vi "NMRfast.vi"() -> ()   [LabVIEW 2013]
uses:
  <vilib>/Utility/file.llb/Read From Spreadsheet File (DBL).vi
  <vilib>/Analysis/NI_AALBase.lvlib
panel:
  out "Diff Sigma":dbl format="%#_13g"
  out "Peak center (MHz)":sgl=213.01303 format="%.3f"
  out "Peak width (MHz)":sgl=0.03243152 format="%.5f"
  in  "Max":bool
  in  "Logoffset (V)":dbl=-5.996000000000003 min=-9.0 max=0.0 step=0.0005 format="%_5g"
  in  "Phase (V)":dbl=6.500000000000002 min=0.0 max=9.0 step=0.0005 format="%_5g"
  out "Telnet error out":errorcluster
  in  "Real/Quad Q curve":bool=TRUE
  out "Temperature (C)":dbl(graph)=26.25
  out "+3V supply":dbl=3.245 format="%_4g"
  out "Temp (C)":dbl=26.25 format="%_4g"
  in  "RemovePed":bool=TRUE
  in  "IF / LOG Det":bool
  in  "Q curve file":string="realback212a.txt"
  out "File name 2":string="C:\\users\\plm\\Desktop\\rssmt\\realback212a.txt"
  in  "AutoTune":bool
  out "RF OK":bool=TRUE
  out "Peak area (V-MHz)":sgl=0.0029111227 format="%.5f"
  in  "Gauss Fit":bool
  out "NMR Graph + Fit":cluster{cluster{dbl, "Numeric":dbl}[]}[](graph)=[{[{212.6, "Numeric"=-0.0034599166666668653}, {212.60999999999999, "Numeric"=-0.0019199166666681458}, {212.62, "Numeric"=-0.0024159166666654327}, {212.63, "Numeric"=-0.0024479166666666894}, {212.64, "Numeric"=-0.002915916666667886}, {212.65, "Numeric"=-0.003319916666665379}, {212.66, "Numeric"=-0.0013599166666665415}, {212.67, "Numeric"=-0.0008359166666676411}, {212.68, "Numeric"=-0.000347916666665349}, {212.69, "Numeric"=-0.00019591666666641475}, {212.7, "Numeric"=-0.0012799166666674225}, {212.71, "Numeric"=-0.001799916666665344}, {212.72, "Numeric"=-0.00205591666666632}, {212.73, "Numeric"=-0.0023479166666672295}, {212.74, "Numeric"=-0.0016759166666680753}, {212.75, "Numeric"=-0.0010399166666662475}, {212.76, "Numeric"=-0.0017399166666670638}, {212.77, "Numeric"=-0.0017759166666678145}, {212.78, "Numeric"=-4.7916666666199086e-05}, {212.79, "Numeric"=-0.000755916666666921}, {212.8, "Numeric"=-0.0004999166666675783}, {212.81, "Numeric"=-0.000479916666666174}, {212.82, "Numeric"=0.00010408333333319572}, {212.82999999999998, "Numeric"=5.208333333263284e-05}, {212.84, "Numeric"=0.0012640833333338224}, {212.85, "Numeric"=0.001440083333333288}, {212.85999999999999, "Numeric"=0.00018008333333281723}, {212.87, "Numeric"=-0.0004159166666662063}, {212.88, "Numeric"=0.00015208333333335388}, {212.89, "Numeric"=-0.0004159166666670216}, {212.9, "Numeric"=8.008333333374331e-05}, {212.91, "Numeric"=0.0012400833333333942}, {212.92, "Numeric"=0.001664083333333114}, {212.93, "Numeric"=0.0014520833333336643}, {212.94, "Numeric"=0.003104083333333411}, {212.95, "Numeric"=0.005720083333333222}, {212.96, "Numeric"=0.01040008333333356}, {212.97, "Numeric"=0.019844083333333404}, {212.98, "Numeric"=0.030252083333333308}, {212.99, "Numeric"=0.03002408333333328}, {213.0, "Numeric"=0.02346008333333337}, {213.01, "Numeric"=0.01956008333333337}, {213.02, "Numeric"=0.017724083333333435}, {213.03, "Numeric"=0.014152083333333312}, {213.04, "Numeric"=0.014044083333333405}, {213.05, "Numeric"=0.015100083333333562}, {213.06, "Numeric"=0.015320083333333224}, {213.07, "Numeric"=0.01620408333333341}, {213.08, "Numeric"=0.013052083333333665}, {213.09, "Numeric"=0.009264083333333114}, {213.1, "Numeric"=0.006440083333333396}, {213.11, "Numeric"=0.005480083333333742}, {213.12, "Numeric"=0.005284083333332979}, {213.13, "Numeric"=0.004852083333333353}, {213.14000000000001, "Numeric"=0.0034840833333337944}, {213.15, "Numeric"=0.002580083333332819}, {213.16, "Numeric"=0.0032400833333332884}, {213.17000000000002, "Numeric"=0.004064083333333823}, {213.18, "Numeric"=0.003452083333332633}, {213.19, "Numeric"=0.003604083333333198}, {213.2, "Numeric"=0.003520083333333825}, {213.21, "Numeric"=0.003500083333332421}, {213.22, "Numeric"=0.0018440833333330771}, {213.23, "Numeric"=0.0016520833333337993}, {213.24, "Numeric"=0.0013240833333345902}, {213.25, "Numeric"=0.00026008333333293627}, {213.26, "Numeric"=0.000760083333333752}, {213.27, "Numeric"=0.0010240833333346388}, {213.28, "Numeric"=0.0006520833333327732}, {213.29, "Numeric"=0.0013440833333336804}, {213.3, "Numeric"=0.0012000833333346552}, {213.31, "Numeric"=0.001420083333332575}, {213.32, "Numeric"=0.0020040833333335823}, {213.33, "Numeric"=0.0020520833333346504}, {213.34, "Numeric"=-0.00013591666666763844}, {213.35, "Numeric"=-0.0009599166666665439}, {213.36, "Numeric"=-0.0002199166666653771}, {213.37, "Numeric"=-0.0004159166666678838}, {213.38, "Numeric"=0.00045208333333330696}, {213.39000000000001, "Numeric"=0.0012840833333345658}, {213.4, "Numeric"=0.0008800833333318511}]}]
  in  "Amp of Q curve":dbl=1.8000000000000034 min=0.0 max=29.0 step=0.01 format="%_3f"
  in  "Subtract Q curve":bool=TRUE
  out "Pedestal Offset":dbl(graph)=0.006135416666666641
  out "Pedestal Difference":dbl(graph)=0.002880166666666909
  out "# Good Spectra":i32=988
  in  "Quality cuts":bool=TRUE
  out "Pedestal OK":bool=TRUE
  out "Sweep #":i32=10
  out "1st Sweep":bool
  out "ADC volts OK":bool=TRUE
  out "Peak Height Distribution":cluster{"Y":dbl[], "Y":dbl[]}[](graph)=[{"Y"=[0.02747215624999998, 0.027537302083333312, 0.027602447916666644, 0.02766759374999998, 0.02773273958333331, 0.027797885416666647, 0.02786303124999998, 0.02792817708333331, 0.027993322916666646, 0.02805846874999998, 0.028123614583333314, 0.028188760416666646, 0.028253906249999978, 0.028319052083333313, 0.028384197916666645, 0.02844934374999998, 0.028514489583333313, 0.028579635416666645, 0.02864478124999998, 0.028709927083333312, 0.028775072916666644, 0.02884021874999998, 0.02890536458333331, 0.028970510416666647, 0.02903565624999998, 0.02910080208333331, 0.029165947916666646, 0.02923109374999998, 0.029296239583333314, 0.029361385416666646, 0.029426531249999978, 0.029491677083333313, 0.029556822916666645, 0.02962196874999998, 0.029687114583333313, 0.029752260416666645, 0.02981740624999998, 0.029882552083333312, 0.029947697916666648, 0.03001284374999998, 0.03007798958333331, 0.030143135416666647, 0.03020828124999998, 0.03027342708333331, 0.030338572916666647, 0.03040371874999998, 0.030468864583333314, 0.030534010416666646, 0.030599156249999978, 0.030664302083333313, 0.030729447916666645, 0.03079459374999998, 0.030859739583333313, 0.030924885416666645, 0.03099003124999998, 0.031055177083333312, 0.031120322916666648, 0.03118546874999998, 0.031250614583333315, 0.031315760416666644, 0.03138090624999998, 0.031446052083333315, 0.03151119791666664, 0.03157634374999998, 0.031641489583333314, 0.03170663541666665, 0.03177178124999998, 0.03183692708333331, 0.03190207291666665, 0.03196721874999998, 0.03203236458333331, 0.03209751041666665, 0.03216265624999998, 0.03222780208333331, 0.03229294791666665, 0.032358093749999976, 0.03242323958333331, 0.03248838541666665, 0.03255353124999998, 0.03261867708333331, 0.03268382291666665, 0.03274896874999998, 0.03281411458333331, 0.032879260416666646, 0.03294440624999998, 0.03300955208333331, 0.033074697916666645, 0.03313984374999998, 0.033204989583333316, 0.033270135416666645, 0.03333528124999998, 0.033400427083333316, 0.033465572916666644, 0.03353071874999998, 0.033595864583333315, 0.033661010416666644, 0.03372615624999998, 0.033791302083333315, 0.03385644791666664, 0.03392159374999998], "Y"=[4.0, 0.0, 0.0, 0.0, 2.0, 1.0, 4.0, 2.0, 4.0, 1.0, 2.0, 3.0, 2.0, 6.0, 3.0, 2.0, 4.0, 7.0, 5.0, 5.0, 11.0, 4.0, 7.0, 6.0, 10.0, 7.0, 10.0, 6.0, 14.0, 16.0, 11.0, 9.0, 13.0, 10.0, 12.0, 17.0, 20.0, 12.0, 18.0, 10.0, 15.0, 13.0, 11.0, 19.0, 21.0, 12.0, 18.0, 21.0, 23.0, 16.0, 24.0, 15.0, 12.0, 17.0, 18.0, 26.0, 22.0, 26.0, 29.0, 17.0, 29.0, 20.0, 16.0, 14.0, 13.0, 13.0, 16.0, 19.0, 12.0, 13.0, 16.0, 6.0, 9.0, 9.0, 11.0, 9.0, 5.0, 9.0, 9.0, 2.0, 10.0, 4.0, 11.0, 10.0, 3.0, 5.0, 3.0, 4.0, 3.0, 6.0, 2.0, 2.0, 3.0, 1.0, 1.0, 4.0, 4.0, 3.0, 1.0, 3.0]}]
  in  "# of Sweeps":i32=1000
  out "S/N":dbl=24.050317766918518 format="%_3g"
  out "Peak mean (V)":dbl=0.030799925016869054 format="%_4g"
  out "Peak Height":dbl(graph)=0.030252083333333308
  in  "Raw Data":bool=TRUE
  in  "Tank RF":bool=TRUE
  in  "IF Atten (dB)":i8=3 min=0 max=31 step=1
  in  "IFoffset (V)":dbl=5.2303410000000135 min=-0.0 max=9.0 step=0.001 format="%.4f"
  in  "Tune  (V)":dbl=0.3670000000000009 min=-0.5 max=8.0 step=0.001 format="%.4f"
  in  "Hi / Lo Gain":bool
  out "Voltage Array":sgl[](array[numeric])=[0.0322, 0.0323, 0.0304, 0.029, 0.0272, 0.0255, 0.0262, 0.0255, 0.0248, 0.0238, 0.0216, 0.02, 0.0187, 0.0174, 0.0171, 0.0168, 0.0152, 0.0143, 0.0152, 0.0137, 0.0132, 0.0125, 0.0124, 0.0117, 0.0123, 0.0119, 0.0101, 0.009, 0.0091, 0.0081, 0.0082, 0.009, 0.0091, 0.0086, 0.01, 0.0124, 0.0169, 0.0262, 0.0365, 0.0362, 0.0296, 0.0257, 0.0239, 0.0204, 0.0204, 0.0216, 0.022, 0.0231, 0.0202, 0.0167, 0.0142, 0.0136, 0.0138, 0.0138, 0.0129, 0.0125, 0.0137, 0.0151, 0.0151, 0.0159, 0.0165, 0.0172, 0.0163, 0.0169, 0.0174, 0.0172, 0.0186, 0.0198, 0.0204, 0.0221, 0.023, 0.0243, 0.026, 0.0272, 0.0262, 0.0266, 0.0286, 0.0297, 0.0319, 0.0341, 0.0351] format="%.4f"
  in  "Invert Polarity":bool=TRUE
  out "Pedestal Diff (V)":sgl=0.0028801668 format="%.3f"
  out "Peak amp (V)":sgl=0.030252084 format="%.3f"
  in  "Save Data to File":bool
  in  "RF Level (dBm)":dbl min=-10.0 max=10.0 step=0.1 format="%.2f"
  out "SMT error out":errorcluster
  out "Sample RMS (V)":dbl=0.0009296296296296295 format="%.4f"
  in  "# Sample/step":i32=80 min=1 max=5000 step=100
  in  "Step Width (MHz)":dbl=0.01 min=0.0 max=1000.0 step=0.0001 format="%.4f"
  in  "Freq Span (MHz)":dbl=0.8 min=0.0 max=3000.0 step=0.1 format="%.3f"
  in  "Center Freq (MHz)":dbl=213.0 min=0.005 max=6000.0 step=0.1 format="%.3f"
  in  "Sweep Mode":u16(ring)=3 items=["Off", "Single", "Auto", "Step"]
  in  "GPIB Addr (28)":refnum<visa-resource-name>="GPIB0::28::INSTR"
  # "E1039 Prototype NMR Control Panel"
  # "Settings"
  # "D\nA\nC"
  # "R\nF\n\nG\nE\nN \n\n+\n\nI\nF"
  # "A\nD\nC"
  # "I\n/\nO"
  # "D\nA\nT\nA\n\nA \nN\nA\nL\nY\nS\nI\nS"
  # "Results"
  # "A\nv\ne\nr\na\ng\ne"
  # "S\nw\ne\ne\np"
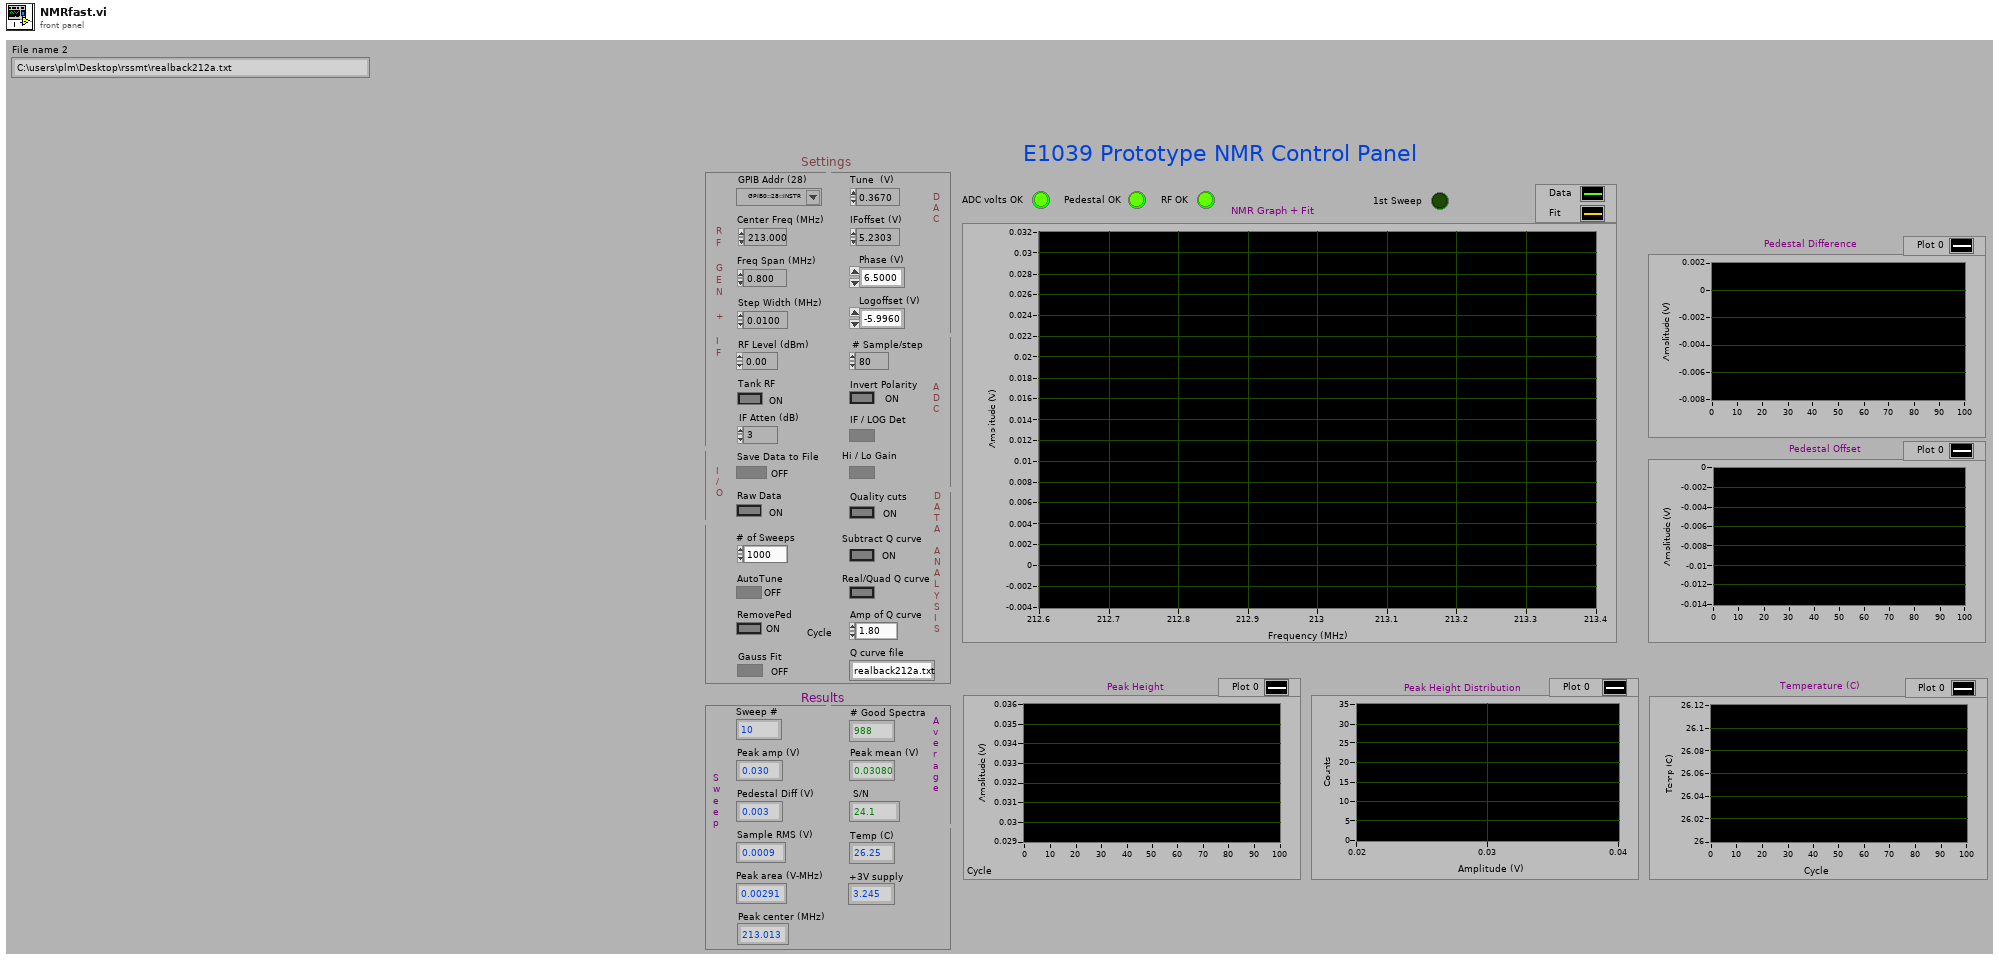
[diagram p1: front panel]
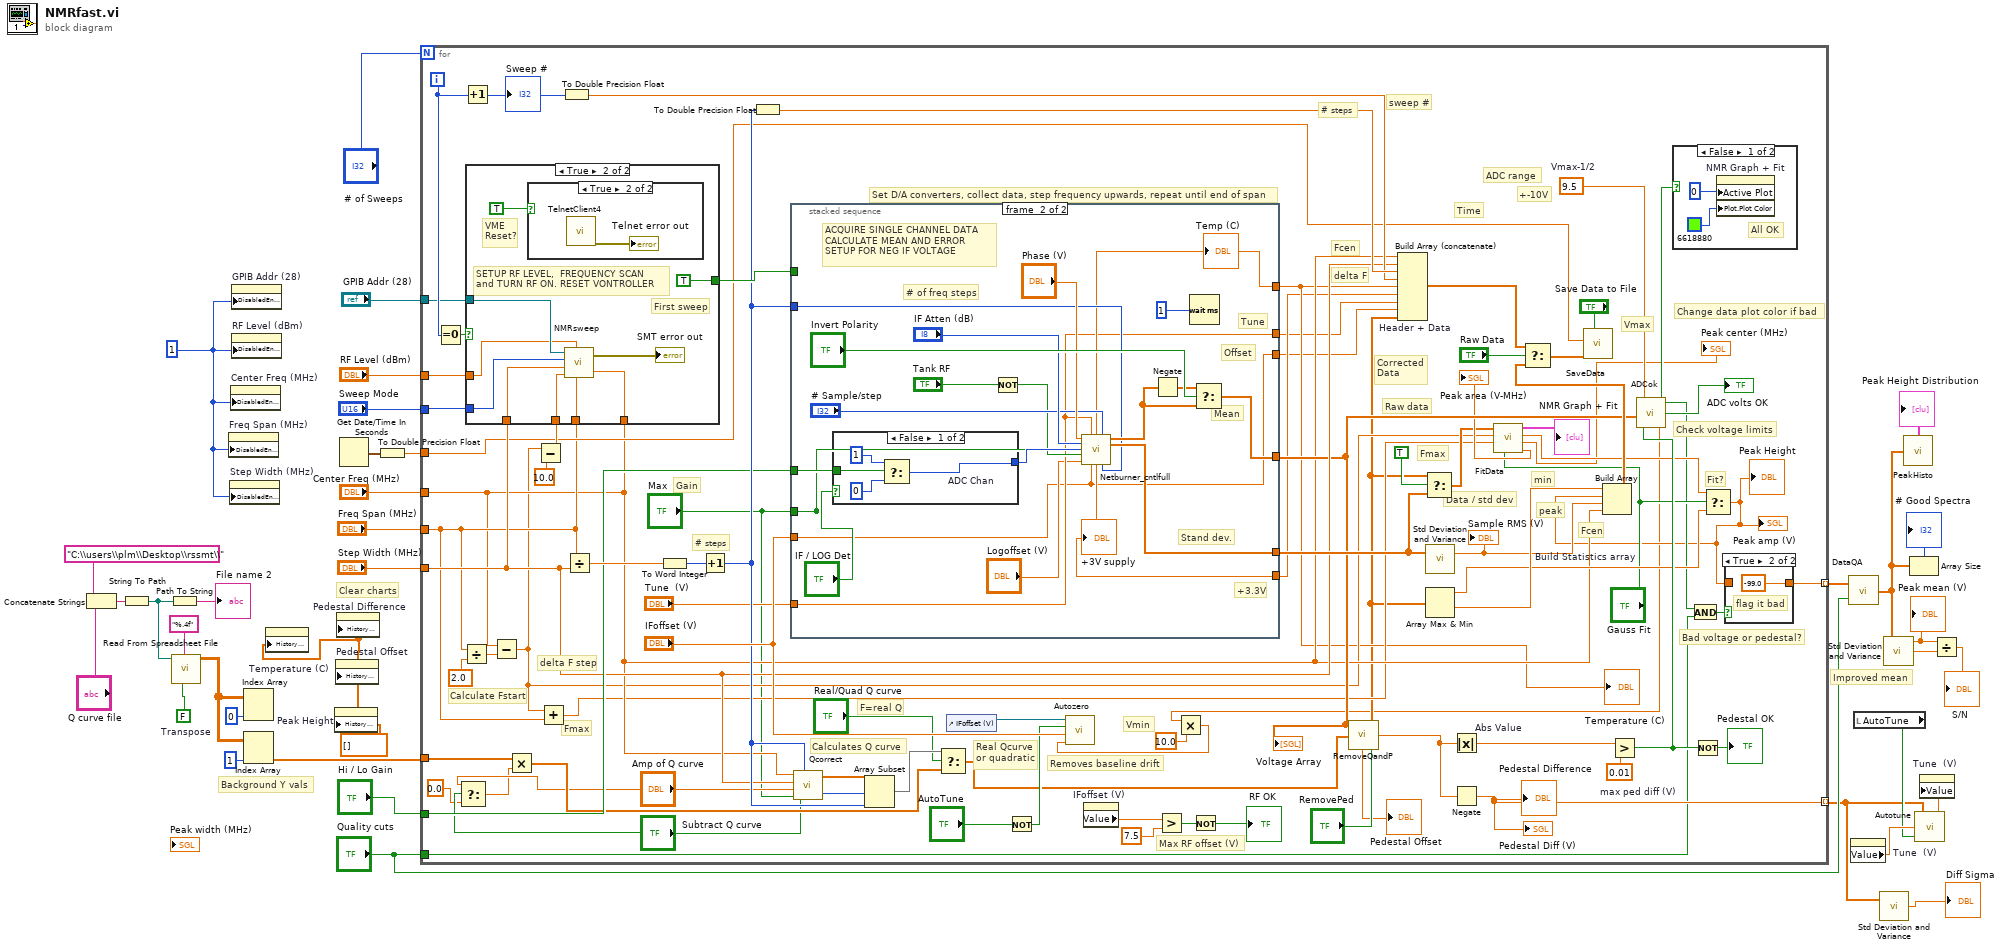
[diagram p0: block diagram]
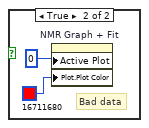
[diagram p2: hidden frame]
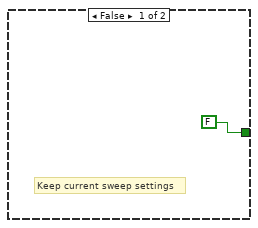
[diagram p4: hidden frame]
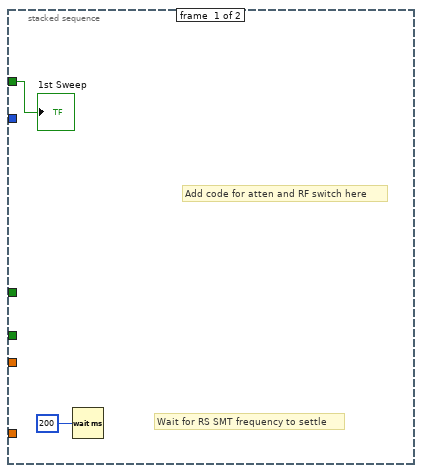
[diagram p6: hidden frame]
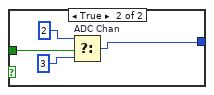
[diagram p7: hidden frame]
diagram:
  w4 = 1
  w16 = FALSE  # Transpose
  w8 = dbl[] []
  # "Background Y vals"
  # "Clear charts"
  # "Improved mean"
  n1 = Concatenate Strings "Concatenate Strings"("C:\\users\\plm\\Desktop\\rssmt\\", "Q curve file") -> (w19:string)
  n2 = String To Path(string=w19) -> (path=w15:path)
  n3 = Path To String(path=w15) -> (string=→"File name 2":string)
  n4 = call-poly <vilib>:"Read From Spreadsheet File.vi"("transpose (no:F)"=w16, "format (%.3f)"="%.4f", "file path (dialog if empty)"=w15) -> ("all rows"=w14:dbl[][])  [unwired: 4 in, 4 out]
  n5 = property on="Freq Span (MHz)" class="DigNum (strict)"("DisabledEnum"=w4) -> ()  [unwired: 2 in, 2 out]
  n6 = property on="Step Width (MHz)" class="DigNum (strict)"("DisabledEnum"=w4) -> ()  [unwired: 2 in, 2 out]
  n7 = property on="Center Freq (MHz)" class="DigNum (strict)"("DisabledEnum"=w4) -> ()  [unwired: 2 in, 2 out]
  n8 = property on="GPIB Addr (28)" class="VISAName"("DisabledEnum"=w4) -> ()  [unwired: 2 in, 2 out]
  n9 = property on="RF Level (dBm)" class="DigNum (strict)"("DisabledEnum"=w4) -> ()  [unwired: 2 in, 2 out]
  n10 = Index Array "Index Array"(array=w14, index (col)=0) -> ()  [unwired: 1 in, 1 out]
  n11 = Index Array(array=w14, index (col)=1) -> (element=w9:dbl[])  [unwired: 1 in]
  n12 = property on="Temperature (C)" class="WFChart (strict)"("History Data"=w8) -> ()  [unwired: 2 in, 2 out]
  n13 = property on="Peak Height" class="WFChart (strict)"("History Data"=w8) -> ()  [unwired: 2 in, 2 out]
  n14 = property on="Pedestal Offset" class="WFChart (strict)"("History Data"=w8) -> ()  [unwired: 2 in, 2 out]
  n15 = property on="Pedestal Difference" class="WFChart (strict)"("History Data"=w8) -> ()  [unwired: 2 in, 2 out]
  n16 = Get Date/Time In Seconds() -> (seconds since 1Jan1904=w21:timestamp)
  n17 = To Double Precision Float(number=w21) -> (double precision float=w20:dbl)
  n18 = for {
    N: "# of Sweeps" -> [_]
    tunnel: [w104] -> w34 mode=indexing
    tunnel: "Quality cuts" -> [w83]
    tunnel: [w88] -> w2 mode=indexing
    tunnel: "Center Freq (MHz)" -> [w70]
    tunnel: "Freq Span (MHz)" -> [w76]
    tunnel: "Step Width (MHz)" -> [w82]
    tunnel: "Sweep Mode" -> [w92]
    tunnel: "Hi / Lo Gain" -> [w91]
    tunnel: "GPIB Addr (28)" -> [w90]
    tunnel: "RF Level (dBm)" -> [w89]
    tunnel: w20 -> [w77]
    tunnel: w9 -> [w55]
    i -> [w102]
    w86 = 9.5  # Vmax-1/2
    w105 = 0.01  # max ped diff (V)
    # "Gain"
    # "F=real Q"
    # "Real Qcurve\nor quadratic"
    # "+-10V"
    # "Vmax"
    # "Change data plot color if bad"
    # "Max RF offset (V)"
    # "Fmax"
    # "Fit?"
    # "Fmax"
    # "Time"
    # "Vmin"
    # "min"
    # "peak"
    # "Raw data"
    # "Corrected\nData"
    # "Fcen"
    # "delta F"
    # "# steps"
    # "ADC range"
    # "sweep #"
    # "Fcen"
    # "Set D/A converters, collect data, step frequency upwards, repeat until end of span"
    # "Calculates Q curve"
    # "Removes baseline drift"
    # "Bad voltage or pedestal?"
    # "Check voltage limits"
    # "Data / std dev"
    # "# steps"
    # "Calculate Fstart"
    # "delta F step"
    n19 = Equal To 0?(x=w102) -> (x = 0?=w107:bool)
    n20 = Select(t="Amp of Q curve", s="Subtract Q curve", f=0.0) -> (s? t:f=w50:dbl)
    n21 = Divide(x=w76, y=sgl 2.0) -> (x/y=w118:dbl)
    n22 = Increment(x=w102) -> (x+1=w93:i32)
    "Sweep #" <- w93
    n23 = Subtract(x=w70, y=w118) -> (x-y=w65:dbl)
    n24 = Multiply(x=w55, y=w50) -> (x*y=w54:dbl[])
    n25 = Subtract(x=w65, y=10.0) -> (x-y=w116:dbl)
    n26 = case shown="True" w107 {
      tunnel: w116 -> [_ w137]
      tunnel: w82 -> [_ w135]
      tunnel: w70 -> [_ w134]
      tunnel: w76 -> [_ w136]
      tunnel: [FALSE TRUE] -> w106
      tunnel: w92 -> [_ w131]
      tunnel: w90 -> [_ w130]
      tunnel: w89 -> [_ w129]
      frame False {
        # "Keep current sweep settings"
      }
      frame True {
        # "VME\nReset?"
        # "First sweep"
        # "SETUP RF LEVEL,  FREQUENCY SCAN\nand TURN RF ON. RESET VONTROLLER"
        n27 = case shown="True" TRUE {
          frame False {
          }
          frame True {
            n28 = call "TelnetClient4.vi"() -> ("Telnet error"=→"Telnet error out":errorcluster)  [unwired: 4 in, 3 out]
          }
        }
        n29 = call "NMRsweep.vi"("Center Freq (MHz)"=w134, "Freq Span (MHz)"=w136, "RF Level (dBm)"=w129, "Foffset (MHz)"=w137, "Step Width (MHz)"=w135, "Sweep Mode"=w131, "GPIB Addr (28)"=w130) -> ("error out"=→"SMT error out":errorcluster)
      }
    }
    n30 = Add(x=w65, y=w76) -> (x+y=w64:dbl)
    n31 = To Double Precision Float(number=w93) -> (double precision float=w94:dbl)
    n32 = Divide(x=w76, y=w82) -> (x/y=w120:dbl)
    n33 = To Word Integer(number=w120) -> (16bit integer=w117:i16)
    n34 = Increment(x=w117) -> (x+1=w96:i16)
    n35 = To Double Precision Float(number=w96) -> (double precision float=w95:dbl)
    n36 = stacked-sequence {
      tunnel: [_ w152] -> w110
      tunnel: [_ w159] -> w80
      tunnel: w96 -> [_ w149]
      tunnel: "IFoffset (V)" -> [_ w142]
      tunnel: w91 -> [_ w157]
      tunnel: w106 -> [w139 _]
      tunnel: "Tune  (V)" -> [_ w144]
      tunnel: [_ w148] -> w46
      tunnel: [_ w145] -> w45
      tunnel: [_ w144] -> w43
      tunnel: [_ w142] -> w42
      tunnel: [_ w141] -> _
      tunnel: "Max" -> [_ w141]
      frame #0 {
        # "Add code for atten and RF switch here"
        # "Wait for RS SMT frequency to settle"
        n37 = Wait (ms)(milliseconds to wait=200) -> ()  [unwired: 1 out]
        "1st Sweep" <- w139
      }
      frame #1 {
        # "+3.3V"
        # "Offset"
        # "Tune"
        # "Stand dev."
        # "Mean"
        # "ACQUIRE SINGLE CHANNEL DATA\nCALCULATE MEAN AND ERROR\nSETUP FOR NEG IF VOLTAGE"
        # "# of freq steps"
        n38 = case shown="False" "IF / LOG Det" {
          tunnel: w157 -> [w165 w166]
          tunnel: [w162 w167] -> w151
          frame False {
            n39 = Select "ADC Chan"(t=1, s=w165, f=0) -> (s? t:f=w162:i32)
          }
          frame True {
            n40 = Select "ADC Chan"(t=2, s=w166, f=3) -> (s? t:f=w167:i32)
          }
        }
        n41 = Not(x="Tank RF") -> (.not. x?=w147:bool)
        n42 = call "Netburner_cntlfull.vi"("Phase Volt"="Phase (V)", "Tune Volt"=w144, "# Data"="# Sample/step", "IF Atten (dB)"="IF Atten (dB)", "NMR ADC"=w151, "Hi Gain"=w141, "Tank RF"=w147, "LogOff Volt"="Logoffset (V)", "IFOff Volt"=w142, "# f steps"=w149) -> ("Temp (C)"=w148:dbl, "ADC value"=w153:dbl[], "ADC error"=w152:dbl[], "Volts"=w145:dbl)  [unwired: 2 out]
        "Temp (C)" <- w148
        "+3V supply" <- w145
        n43 = Negate(x=w153) -> (-x=w158:dbl[])
        n44 = Wait (ms)(milliseconds to wait=1) -> ()  [unwired: 1 out]
        n45 = Select(t=w158, s="Invert Polarity", f=w153) -> (s? t:f=w159:dbl[])
      }
    }
    "Voltage Array" <- w80
    "Temperature (C)" <- w46
    n46 = call "Qcorrect.vi"("Subtract Q curve"="Subtract Q curve", "Nstep"=w96, "Max Gain"="Max", "Amp of Q curve"="Amp of Q curve", "Step Width (MHz)"=w82, "Center Freq (MHz)"=w70) -> ("Start"=w111:i32, "Array"=w112:dbl[])
    n47 = Array Subset "Array Subset"(array=w112, index=w111, length=w96) -> (w58:dbl[])
    n48 = Select(t=w58, s="Real/Quad Q curve", f=w54) -> (s? t:f=w57:dbl[])
    n49 = control-ref of="IFoffset (V)"() -> (w85:refnum<vi>)
    n50 = Not(x="AutoTune") -> (.not. x?=w59:bool)
    n51 = property on="IFoffset (V)" class="DigNum (strict)"() -> ("Value"=w74:dbl)  [unwired: 2 in, 2 out]
    n52 = Greater?(x=w74, y=7.5) -> (0:w72:bool)
    n53 = Not(x=w72) -> (.not. x?=→"RF OK":bool)
    n54 = call "RemoveQandP.vi"("Subtract Ped?"="RemovePed", "Qcurve"=w57, "Raw data"=w80) -> ("Ped L-R"=w98:dbl, "Corrected data"=w44:dbl[], "Ped Offfset"=→"Pedestal Offset":dbl)
    n55 = Build Array (concatenate) "Header + Data"(w70, w82, w95, w94, w46, w45, w43, w42, w44) -> (w97:dbl[])
    n56 = Select(t=w44, s=TRUE, f=w110) -> (s? t:f=w66:dbl[])
    n57 = call <vilib>:"Std Deviation and Variance.vi"("X"=w110) -> ("mean"=w81:dbl)  [unwired: 1 in, 2 out]
    "Sample RMS (V)" <- w81
    n58 = Array Max & Min(array=w44) -> (max value=w75:dbl, min value=w109:dbl)  [unwired: 2 out]
    n59 = Absolute Value "Abs Value"(x=w98) -> (abs(x)=w100:dbl)
    n60 = Negate(x=w98) -> (-x=w88:dbl)
    "Pedestal Diff (V)" <- w88
    "Pedestal Difference" <- w88
    n61 = call "FitData.vi"("Fit?"="Gauss Fit", "Fmax"=w64, "Fmin"=w65, "Yarray"=w66) -> ("Peak Area (V-MHz)"=→"Peak area (V-MHz)":dbl, "Center Freq (MHz)"=→"Peak center (MHz)":dbl, "Amplitude (V)"=w68:dbl, "NMR Graph + Fit"=→"NMR Graph + Fit":cluster{cluster{dbl, "Numeric":dbl}[]}[])  [unwired: 1 out]
    n62 = Greater?(x=w100, y=w105) -> (0:w87:bool)
    n63 = call "ADCok.vi"("PedOK"=w87, "Array"=w80, "Vmax-1/2"=w86) -> ("Vmin"=w39:dbl, "ADC voltages OK"=→"ADC volts OK":bool, "Allok"=w62:bool)
    n64 = Multiply(x=w39, y=10.0) -> (x*y=w37:dbl)
    n65 = call "Autozero.vi"("Vmin (V)"=w37, "IFoffset (V)"="IFoffset (V)", "Enable"=w59, "reference"=w85) -> ()
    n66 = case shown="False" w62 {
      frame False {
        # "All OK"
        n67 = property on="NMR Graph + Fit" class="XYGraph (strict)"("Active Plot"=0, "Plot.Plot Color"=u32 6618880) -> ()  [unwired: 2 in, 2 out]
      }
      frame True {
        # "Bad data"
        n68 = property on="NMR Graph + Fit" class="XYGraph (strict)"("Active Plot"=0, "Plot.Plot Color"=u32 16711680) -> ()  [unwired: 2 in, 2 out]
      }
    }
    n69 = And(x=w62, y=w83) -> (x .and. y?=w101:bool)
    n70 = Not(x=w87) -> (.not. x?=→"Pedestal OK":bool)
    n71 = Select(t=w68, s="Gauss Fit", f=w75) -> (s? t:f=w61:dbl)
    "Peak amp (V)" <- w61
    "Peak Height" <- w61
    n72 = Build Array "Build Statistics array"(w109, w61, w81, w70) -> (w115:dbl[])
    n73 = Select(t=w97, s="Raw Data", f=w115) -> (s? t:f=w78:dbl[])
    n74 = call "SaveData.vi"("Array"=w78, "Save Data to File"="Save Data to File", "Ext time (sec)"=w77) -> ()  [unwired: 1 out]
    n75 = case shown="True" w101 {
      tunnel: [w125 -99.0] -> w104
      tunnel: w61 -> [w125 _]
      frame False {
        # "Data OK"
      }
      frame True {
        # "flag it bad"
      }
    }
  }
  n76 = call "DataQA.vi"("Quality cuts"="Quality cuts", "Data In"=w34) -> ("Data Out"=w33:dbl[])
  n77 = property on="Tune  (V)" class="DigNum (strict)"() -> ("Value"=w24:dbl)  [unwired: 2 in, 2 out]
  n78 = local read "AutoTune"() -> (w3:bool)
  n79 = call <vilib>:"Std Deviation and Variance.vi"("X"=w2) -> ("standard deviation"=→"Diff Sigma":dbl)  [unwired: 1 in, 2 out]
  n80 = call <vilib>:"Std Deviation and Variance.vi"("X"=w33) -> ("mean"=w7:dbl, "standard deviation"=w6:dbl)  [unwired: 1 in, 1 out]
  "Peak mean (V)" <- w7
  n81 = call "PeakHisto.vi"("Data Out"=w33) -> ("XY Graph"=→"Peak Height Distribution":cluster{"Y":dbl[], "Y":dbl[]}[])
  n82 = Array Size(array=w33) -> (size(s)=→"# Good Spectra":i32)
  n83 = call "Autotune.vi"("Adjust Tune"=w3, "Tune Vin"=w24, "Pedestal Diff"=w2) -> ("Tune Vout"=w23:dbl)
  n84 = property on="Tune  (V)" class="DigNum (strict)"("Value"=w23) -> ()  [unwired: 2 in, 2 out]
  n85 = Divide(x=w7, y=w6) -> (x/y=→"S/N":dbl)
